vi "Subtract (Float).vi"(8 "Input Valid":bool, 10 "b":fxp<+,32,32>, 11 "a":fxp<+,32,32>) -> (0 "Output Valid":bool, 3 "a-b":fxp<+,32,32>)   [LabVIEW 2011]
doc: "This VI performs single precision floating point add.\n\n<b> Latency = 11 Ticks </b>"
uses:
  <vilib>/rvi/IPIntegrationNode/IPINode_Utilities/niFpgaIPINodeSimCore.vi
  <vilib>/rvi/FXPMathLib/basic elements/FxpDiscreteDelay/XNode/nifxpmath_DiscreteDelay.xnode
  <vilib>/rvi/XilinxIP/XIPIN_XNode/niFpgaXIPIN.xnode
  <userlib>/FPGA Library/Code Development/SGL/Subtract Float/Subtract Float/SubtractSGL_34DE1114432A912CF86F2DA4B4349472.dll
  <vilib>/rvi/IPIntegrationNode/IPINode_Xnode/niFpgaIPINode.xnode
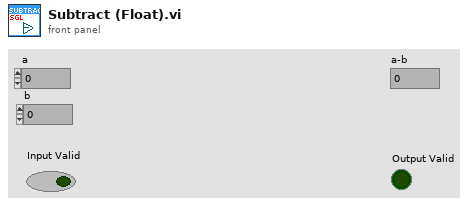
[diagram p1: front panel]
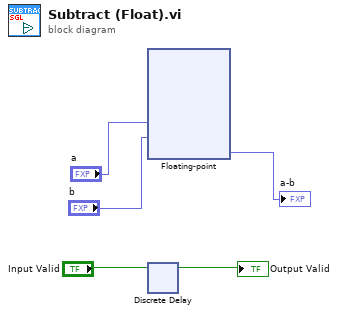
[diagram p0: block diagram]
diagram:
  n1 = xnode ("Floating-point")("a"="a", "b"="b") -> ("result"=→"a-b":fxp<+,32,32>)
  n2 = xnode "Discrete Delay"("D"="Input Valid") -> ("Q"=→"Output Valid":bool)
